vi "SysLog dir select cRIO.vi"(10 "filter":string caption="Filter", 11 "dir list":string[](array[string])) -> (3 "selected filename":string)   [LabVIEW 2020, in "SysLog.lvlib"]
uses:
  SysLog.lvlib
  Sprachverwaltung/FGV Aktion Tabelle zerlegen.ctl
  Sprachverwaltung/Sprachverwaltung.lvlib
  Allgemein/allgemeine Sub-VIs.lvlib
panel:
  in  "Listenfeld":i32(listbox)
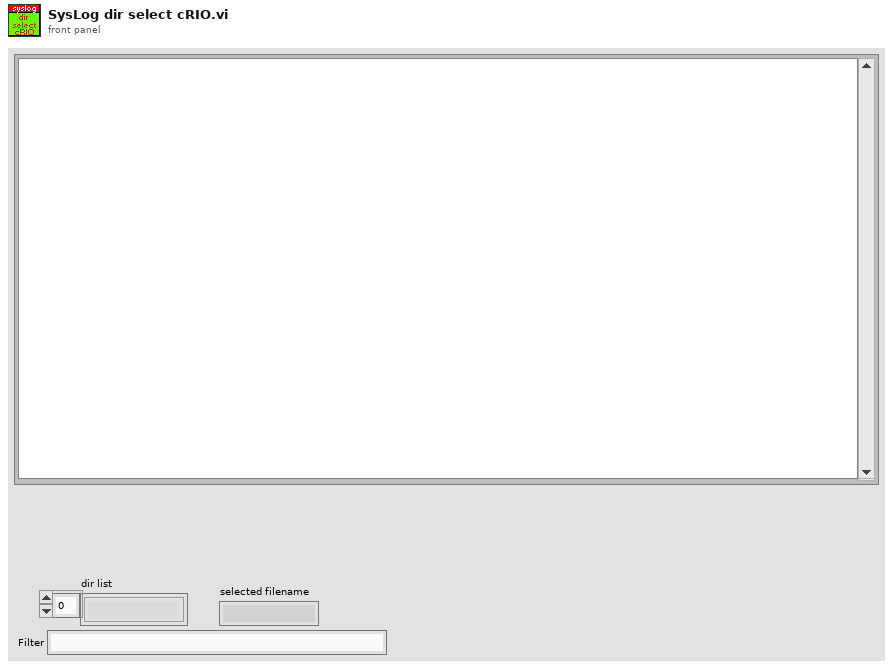
[diagram p1: front panel]
types:
  T1 = typedef "Sprachverwaltung.lvlib/FGV Aktion Tabelle zerlegen.ctl" = enum16{"laden", "vereinzeln", "speichern"}
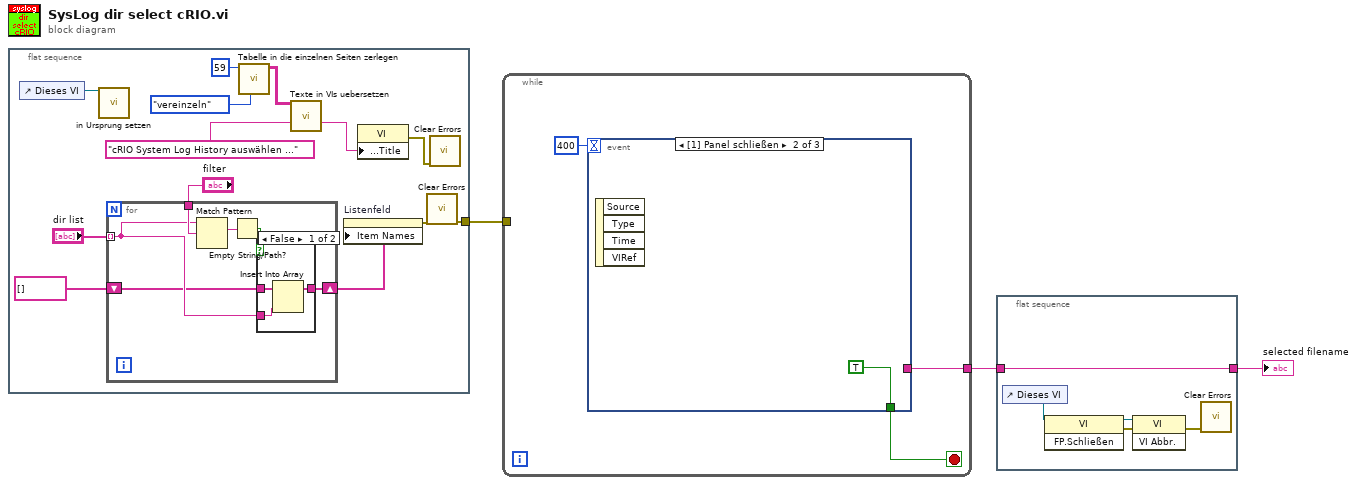
[diagram p0: block diagram]
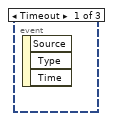
[diagram p2: hidden frame]
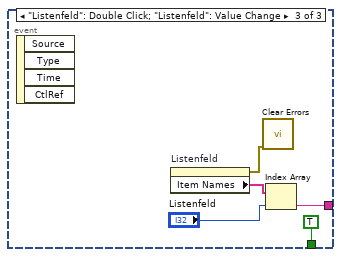
[diagram p3: hidden frame]
diagram:
  n1 = flat-sequence {
    tunnel: [w15] -> w3
    frame #0 {
      n2 = control-ref of="Dieses VI"() -> (w6:refnum<vi>)
      n3 = call "in Ursprung setzen.vi"("VI Referenz"=w6) -> ()  [unwired: 10 in, 1 out]
      n4 = for {
        tunnel: "dir list" -> [w19] mode=indexing
        tunnel: "filter" -> [w22]
        shift-right: [w17] -> w7
        shift-left: string[] [] -> [w18]
        n5 = Match Pattern(string=w19, regular expression=w22) -> (match substring=w21:string)  [unwired: 1 in, 3 out]
        n6 = Empty String/Path?(string/path=w21) -> (empty?=w20:bool)
        n7 = case shown="False" w20 {
          tunnel: w19 -> [w24 _]
          tunnel: w18 -> [w25 w26]
          tunnel: [w23 w26] -> w17
          frame False {
            n8 = Insert Into Array(array=w25, new element=w24) -> (w23:string[])  [unwired: 1 in]
          }
          frame True {
          }
        }
      }
      n9 = call "Tabelle in die einzelnen Seiten zerlegen.vi"("Aktion"=FGV_Aktion_Tabelle_zerlegen."vereinzeln", "Index (Seite)"=59) -> ("Sprachliste"=w11:string[][])  [unwired: 7 in, 2 out]
      n10 = call "Texte in VIs uebersetzen.vi"("Sprachliste"=w11, "String zum Übersetzen"="cRIO System Log History auswählen ..." ("Eingabeaufforderung")) -> ("String zum Übersetzen"=w9:string)  [unwired: 9 in, 4 out]
      n11 = property on="Listenfeld" class="Listenfeld (strikt)"("Item Names"=w7) -> (error out=w16:errorcluster)  [unwired: 2 in, 1 out]
      n12 = property class="VI"("Front Panel.Title"=w9) -> (error out=w13:errorcluster)  [unwired: 2 in, 1 out]
      n13 = call <vilib>:"Clear Errors.vi"("error in (no error)"=w16) -> ("error out"=w15:errorcluster)  [unwired: 5 in, 1 out]
      n14 = call <vilib>:"Clear Errors.vi"("error in (no error)"=w13) -> ()  [unwired: 5 in, 2 out]
    }
  }
  n15 = while {
    tunnel: w3 -> [_]
    tunnel: [w27] -> w2
    stop <- w28 stop-if-true
    n16 = event shown="[1] Panel schließen" {
      selector: _ -> [_ _ _]
      dyn-events: _ -> [_ _ _]
      timeout: 400 -> [_ _ _]
      tunnel: [_ TRUE TRUE] -> w28
      tunnel: [_ _ w33] -> w27
      event Timeout {
        n17 = event-data() -> ()  [unwired: 1 in, 3 out]
      }
      event Panel Close {
        n18 = event-data() -> ()  [unwired: 1 in, 4 out]
      }
      event "Listenfeld": Double Click; "Listenfeld": Value Change {
        n19 = event-data() -> ()  [unwired: 1 in, 4 out]
        n20 = property on="Listenfeld" class="Listenfeld (strikt)"() -> (error out=w32:errorcluster, "Item Names"=w35:string[])  [unwired: 2 in, 1 out]
        n21 = call <vilib>:"Clear Errors.vi"("error in (no error)"=w32) -> ()  [unwired: 5 in, 2 out]
        n22 = Index Array(array=w35, index="Listenfeld") -> (element=w33:string)
      }
    }
  }
  n23 = flat-sequence {
    tunnel: [w37] -> w1
    tunnel: w2 -> [w37]
    frame #0 {
      n24 = control-ref of="Dieses VI"() -> (w36:refnum<vi>)
      n25 = invoke class="VI" method="FP.Schließen"(reference=w36) -> (reference out=w40:refnum<vi>, error out=w39:errorcluster)  [unwired: 2 in, 1 out]
      n26 = invoke class="VI" method="VI Abbr."(reference=w40, error in=w39) -> (error out=w38:errorcluster)  [unwired: 1 in, 2 out]
      n27 = call <vilib>:"Clear Errors.vi"("error in (no error)"=w38) -> ()  [unwired: 5 in, 2 out]
    }
  }
  "selected filename" <- w1
